vi "计算正图像筛选门限.vi"(1 "差分计算一维矩阵":dbl[](array[numeric]), 2 "少量采样数据量":i32) -> (0 "正图像筛选门限":dbl)   [LabVIEW 2018]
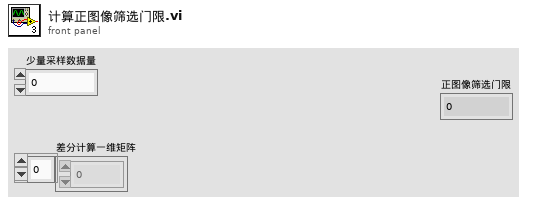
[diagram p1: front panel]
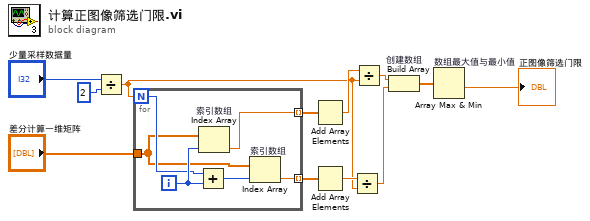
[diagram p0: block diagram]
diagram:
  n1 = Divide(x="少量采样数据量", y=2) -> (x/y=w2:dbl)
  n2 = for {
    N: w2 -> [w17]
    tunnel: "差分计算一维矩阵" -> [w15]
    tunnel: [w14] -> w7 mode=indexing
    tunnel: [w13] -> w4 mode=indexing
    i -> [w18]
    n3 = Add(x=w17, y=w18) -> (x+y=w16:i32)
    n4 = Index Array "索引数组"(array=w15, index=w18) -> (element=w14:dbl)
    n5 = Index Array "索引数组"(array=w15, index=w16) -> (element=w13:dbl)
  }
  n6 = Add Array Elements(numeric array=w7) -> (sum=w6:dbl)
  n7 = Add Array Elements(numeric array=w4) -> (sum=w3:dbl)
  n8 = Divide(x=w3, y=w2) -> (x/y=w1:dbl)
  n9 = Divide(x=w6, y=w2) -> (x/y=w5:dbl)
  n10 = Build Array "创建数组"(w5, w1) -> (w9:dbl[])
  n11 = Array Max & Min "数组最大值与最小值"(array=w9) -> (min value=→"正图像筛选门限":dbl)  [unwired: 3 out]
